vi "Generic Password Dialog.vi"(0 "Enable":bool=TRUE, 3 "Message to Display":string, 5 "error in (no error)":errorcluster) -> (17 "Password:out":string caption="Password:", 18 "OK":bool=TRUE, 19 "error out":errorcluster)   [LabVIEW 2018]
doc: "Displays a standard dialog box that prompts users to enter information, such as a user name and password.\n--------------------\n\nThis Express VI is configured as follows:\n\nMessage to Display to the User:Enter password to unlock server...\nThe inputs are: \nText Entry Box: Password:"
uses:
  <vilib>/event_ctls.llb/eventvkey.ctl
panel:
  in  "Password:":string
  out "String":string
  in  "Cancel":bool
  in  "OK2":bool
  in  "OK1":bool
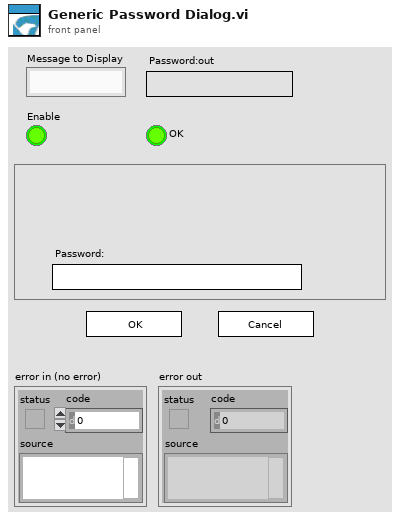
[diagram p1: front panel]
types:
  T1 = cluster{"Input Name":string, "Input Data Type":i32}[]
  T2 = typedef "eventvkey.ctl" = enum16{"ASCII", "Enter", "Return", "Shift", "Ctrl", "Alt", "Cmd", "Opt", "Caps", "NumLock", "Clear", "Break", "Up", "Down", "Left", "Right", "Insert", "Delete", "Home", "End", "PageUp", "PageDown", "Escape", "Help", "Pause", "ScrollLock", "F1", "F2", "F3", "F4", "F5", "F6", "F7", "F8", "F9", "F10", "F11", "F12", "F13", "F14", "F15", "F16", "F17", "F18", "F19", "F20", "F21", "F22", "F23", "F24", "Play", "VolumeUp", "VolumeDown", "Mute", "Two Byte Char"}
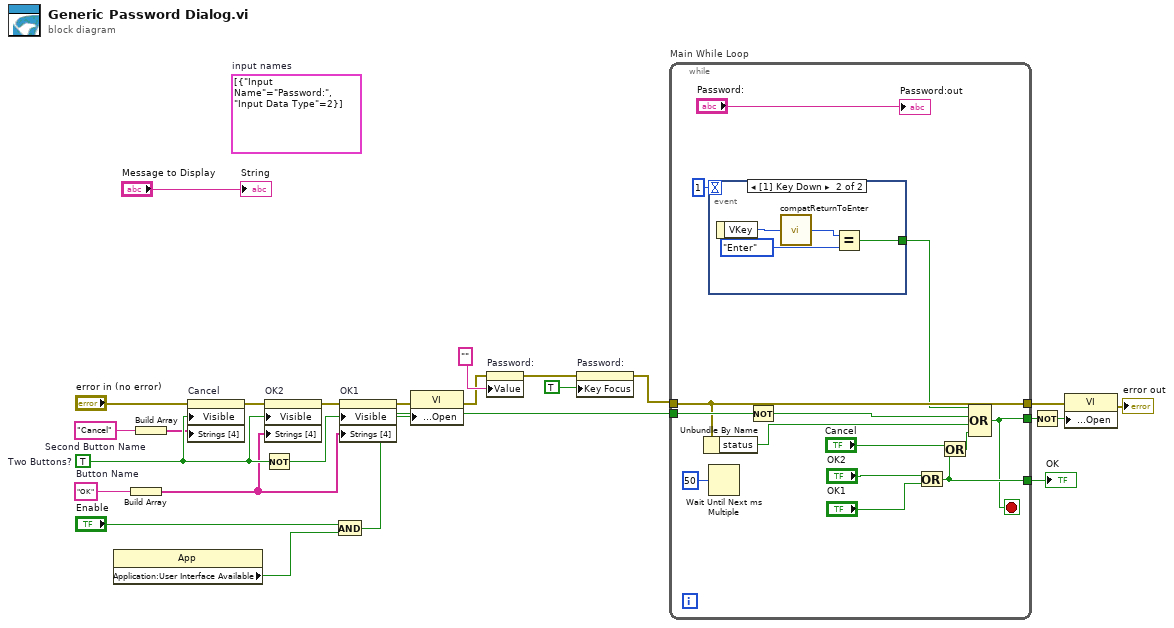
[diagram p0: block diagram]
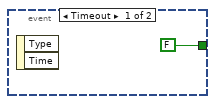
[diagram p2: hidden frame]
diagram:
  (unwired) T1 [{"Input Name"="Password:", "Input Data Type"=2}]  # input names
  w16 = "Cancel"  # Second Button Name
  w14 = "OK"  # Button Name
  w24 = TRUE  # Two Buttons?
  n1 = property class="App"() -> ("Application:User Interface Available"=w7:bool)  [unwired: 2 in, 2 out]
  n2 = Build Array(w14) -> (w15:string[])
  n3 = Build Array(w16) -> (w17:string[])
  n4 = property on="Cancel" class="Bool"(error in="error in (no error)", "Visible"=w24, "Strings [4]"=w17) -> (error out=w21:errorcluster)  [unwired: 1 in, 1 out]
  n5 = Not(x=w24) -> (.not. x?=w22:bool)
  n6 = property on="OK2" class="Bool"(error in=w21, "Visible"=w24, "Strings [4]"=w15) -> (error out=w20:errorcluster)  [unwired: 1 in, 1 out]
  n7 = And(x="Enable", y=w7) -> (x .and. y?=w8:bool)
  n8 = property on="OK1" class="Bool"(error in=w20, "Visible"=w22, "Strings [4]"=w15) -> (error out=w13:errorcluster)  [unwired: 1 in, 1 out]
  n9 = property class="VI"(error in=w13, "Front Panel Window:Open"=w8) -> (error out=w2:errorcluster)  [unwired: 1 in, 1 out]
  n10 = property on="Password:" class="Str"(error in=w2, "Value"="" ("Password:")) -> (error out=w1:errorcluster)  [unwired: 1 in, 1 out]
  n11 = property on="Password:" class="Str"(error in=w1, "Key Focus"=TRUE) -> (error out=w5:errorcluster)  [unwired: 1 in, 1 out]
  n12 = while "Main While Loop" {
    tunnel: [w35] -> w23
    tunnel: w8 -> [w34]
    tunnel: [w32] -> w18
    tunnel: w5 -> [w31]
    tunnel: [w31] -> w11
    stop <- w32 stop-if-true
    n13 = Unbundle By Name(w31) -> ("status"=w29:bool)
    n14 = event shown="[1] Key Down" {
      selector: _ -> [_ _]
      dyn-events: _ -> [_ _]
      timeout: 1 -> [_ _]
      tunnel: [FALSE w41] -> w25
      event Timeout {
        n15 = event-data() -> ()  [unwired: 1 in, 2 out]
      }
      event Key Down {
        n16 = event-data() -> ("VKey"=w40:T2)  [unwired: 1 in]
        n17 = call <vilib>:"compatReturnToEnter.vi"("VKey"=w40) -> ("VKey"=w42:T2)
        n18 = Equal?(x=w42, y=eventvkey."Enter" ("VKey")) -> (x = y?=w41:bool)
      }
    }
    n19 = Wait Until Next ms Multiple(millisecond multiple=u32 50) -> ()  [unwired: 1 out]
    n20 = Not(x=w34) -> (.not. x?=w33:bool)
    n21 = Or(x="OK2", y="OK1") -> (x .or. y?=w35:bool)
    n22 = Or(x="Cancel", y=w35) -> (x .or. y?=w30:bool)
    n23 = Compound Arithmetic op=OR(w25, w33, w29, w30) -> (w32:bool)
    "Password:out" <- "Password:"
  }
  "OK" <- w23
  n24 = Not(x=w18) -> (.not. x?=w19:bool)
  n25 = property class="VI"(error in=w11, "Front Panel Window:Open"=w19) -> (error out=→"error out":errorcluster)  [unwired: 1 in, 1 out]
  "String" <- "Message to Display"
